vi "UnboxPath.vi"(10 "Path in":refnum<class "Path.lvclass">) -> (2 "Path":path)   [LabVIEW 2013, in "LapDog.Collections.v1.Common.lvlib" / "Path.lvclass"]
uses:
  Path.lvclass
  Path.lvclass/Path.ctl
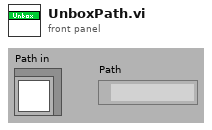
[diagram p1: front panel]
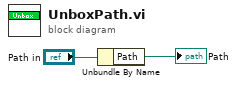
[diagram p0: block diagram]
diagram:
  n1 = Unbundle By Name("Path in") -> ("Path"=→"Path":path)
